vi "Resample XY Array.vi"(8 "error in (no error)":errorcluster, 10 "Fs":dbl, 11 "XY [] in":cluster{dbl[], dbl[]}[](array[cluster])) -> (0 "error out":errorcluster, 3 "XY [] out":cluster{"X-array":dbl[], "Y-array":dbl[]}[](array[cluster]))   [LabVIEW 2016, in "Transport.lvclass"]
uses:
  Transport.lvclass
  <vilib>/measure/maresamp.llb/Resample Pair of Arrays (single shot).vi
  <vilib>/measure/NI_MAPro.lvlib
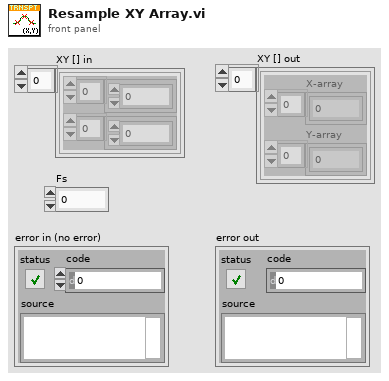
[diagram p1: front panel]
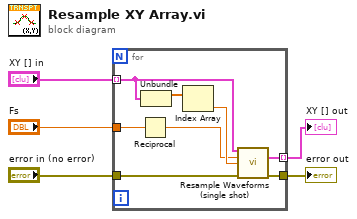
[diagram p0: block diagram]
diagram:
  n1 = for {
    tunnel: "XY [] in" -> [w11] mode=indexing
    tunnel: [w10] -> w2 mode=indexing
    tunnel: "Fs" -> [w8]
    tunnel: "error in (no error)" -> [w7]
    tunnel: [w6] -> w5
    n2 = Reciprocal(x=w8) -> (1/x=w9:dbl)
    n3 = Unbundle(w11) -> (w13:dbl[])  [unwired: 1 out]
    n4 = Index Array(array=w13) -> (element=w12:dbl)  [unwired: 1 in]
    n5 = call-poly <vilib>:"Resample Waveforms (single shot).vi"("XY-data in"=w11, "dt"=w9, "t0"=w12, "error in (no error)"=w7) -> ("XY-data out"=w10:cluster{"X-array":dbl[], "Y-array":dbl[]}, "error out"=w6:errorcluster)  [unwired: 7 in, 3 out]
  }
  "error out" <- w5
  "XY [] out" <- w2
